vi "getShifts.vi"(8 "error in (no error)":errorcluster, 11 "Shift Schedule in":refnum<class "Shift Schedule.lvclass">) -> (0 "error out":errorcluster, 2 "shifts":refnum<class "Shift.lvclass">[](array[class]), 3 "Shift Schedule out":refnum<class "Shift Schedule.lvclass">)   [LabVIEW 2013, in "Shift Schedule.lvclass"]
uses:
  Shift Schedule.lvclass
  Shift.lvclass
  Shift Schedule.lvclass/Shift Schedule.ctl
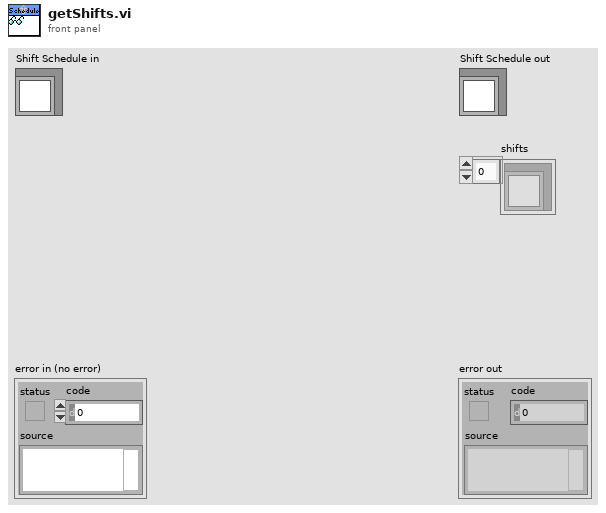
[diagram p1: front panel]
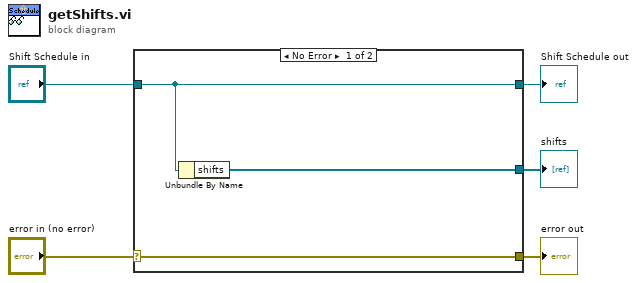
[diagram p0: block diagram]
diagram:
  n1 = case shown="No Error" "error in (no error)" {
    selector: "error in (no error)" -> [w8 w9]
    tunnel: [w8 w9] -> w4
    tunnel: [w7 w10] -> w2
    tunnel: "Shift Schedule in" -> [w7 w10]
    tunnel: [w6 _] -> w1
    frame No Error {
      n2 = Unbundle By Name(w7) -> ("shifts"=w6:refnum<class "Shift.lvclass">[])
    }
    frame Error {
    }
  }
  "error out" <- w4
  "Shift Schedule out" <- w2
  "shifts" <- w1
